vi "reduce golden interval.vi"(8 "error in (no error)":errorcluster, 11 "Autofocus in":refnum<class "Autofocus.lvclass">) -> (0 "error out":errorcluster, 3 "Autofocus out":refnum<class "Autofocus.lvclass">)   [LabVIEW 2012, in "Autofocus.lvclass"]
uses:
  Autofocus.lvclass
  Autofocus.lvclass/Autofocus.ctl
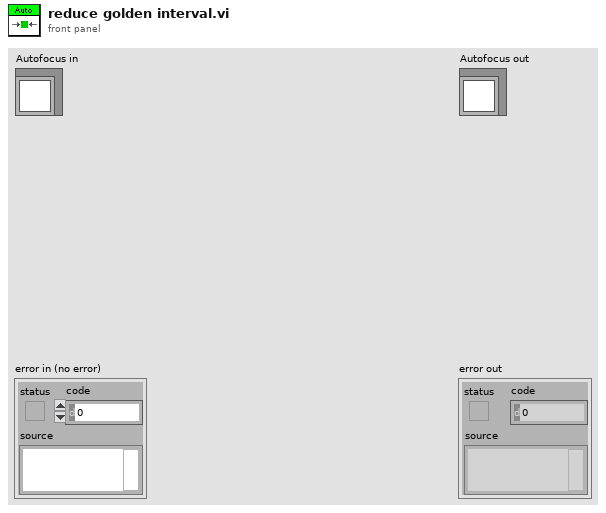
[diagram p1: front panel]
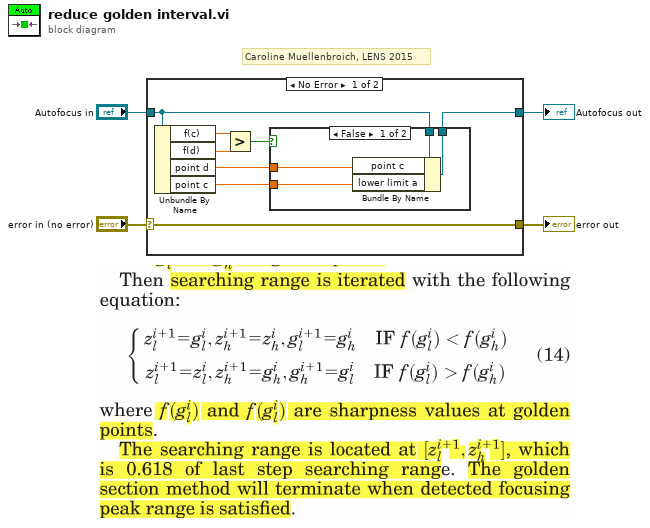
[diagram p0: block diagram]
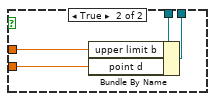
[diagram p2: hidden frame]
diagram:
  # "Caroline Muellenbroich, LENS 2015"
  n1 = case shown="No Error" "error in (no error)" {
    selector: "error in (no error)" -> [w12 w22]
    tunnel: [w12 w22] -> w3
    tunnel: [w8 w21] -> w1
    tunnel: "Autofocus in" -> [w9 w21]
    frame No Error {
      n2 = Unbundle By Name(w9) -> ("f(c)"=w11:dbl, "f(d)"=w7:dbl, "point d"=w6:dbl, "point c"=w5:dbl)
      n3 = Greater?(x=w11, y=w7) -> (0:w10:bool)
      n4 = case shown="False" w10 {
        tunnel: w9 -> [w16 w20]
        tunnel: [w15 w19] -> w8
        tunnel: w6 -> [w13 w18]
        tunnel: w5 -> [w14 w17]
        frame False {
          n5 = Bundle By Name(cluster=w16, "point c"=w13, "lower limit a"=w14) -> (w15:refnum<class "Autofocus.lvclass">)
        }
        frame True {
          n6 = Bundle By Name(cluster=w20, "upper limit b"=w18, "point d"=w17) -> (w19:refnum<class "Autofocus.lvclass">)
        }
      }
    }
    frame Error {
    }
  }
  "error out" <- w3
  "Autofocus out" <- w1
